vi "ReadSpectrum(SubVI).vi"(8 "Continuous \nStrobe Delay":i32, 11 "Enter the \nInetegration Time":i32) -> (1 "Spectrum Values":dbl[](array[numeric]), 2 "WL Values":dbl[](array[numeric]), 3 "Number of Spectrometers":i32)   [LabVIEW 2022 SP3]
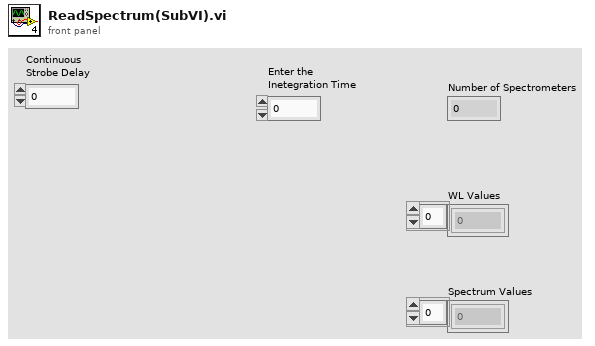
[diagram p1: front panel]
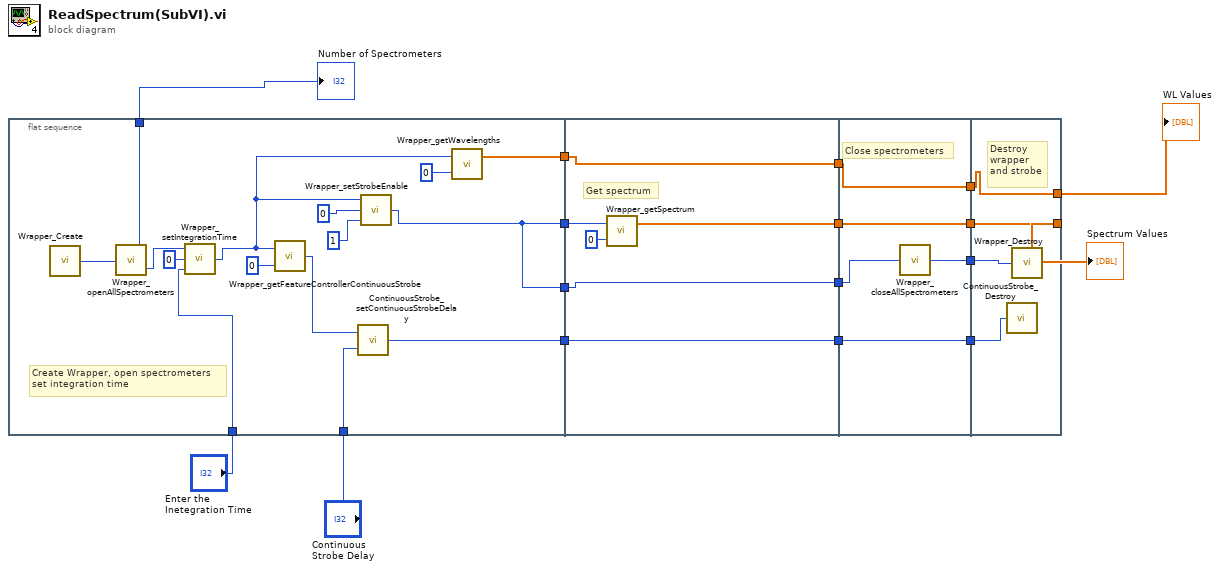
[diagram p0: block diagram]
diagram:
  n1 = flat-sequence {
    tunnel: [w23] -> w17
    tunnel: [w22] -> w16
    tunnel: [w22] -> w15
    tunnel: [w21] -> w14
    tunnel: "Enter the \nInetegration Time" -> [w20]
    tunnel: [w19] -> w5
    tunnel: "Continuous \nStrobe Delay" -> [w18]
    tunnel: [w38] -> w13
    tunnel: w17 -> [w38]
    tunnel: w16 -> [w37]
    tunnel: w15 -> [w35]
    tunnel: [w35] -> w12
    tunnel: w14 -> [w34]
    tunnel: [w34] -> w11
    tunnel: [w33] -> w10
    tunnel: [w43] -> w9
    tunnel: w13 -> [w43]
    tunnel: w12 -> [w42]
    tunnel: [w41] -> w8
    tunnel: [w40] -> w7
    tunnel: w11 -> [w40]
    tunnel: [w39] -> w6
    tunnel: w10 -> [w39]
    tunnel: w9 -> [w47]
    tunnel: w8 -> [w46]
    tunnel: [w45] -> w3
    tunnel: w7 -> [w45]
    tunnel: [w44] -> w2
    tunnel: w6 -> [w44]
    frame #0 {
      # "Create Wrapper, open spectrometers\nset integration time"
      n2 = call "Wrapper_Create.vi"() -> ("Wrapper"=w32:u32)
      n3 = call "Wrapper_openAllSpectrometers.vi"("Wrapper In"=w32) -> ("Number of Spectrometers"=w19:i32, "Wrapper Out"=w26:u32)
      n4 = call "Wrapper_setIntegrationTime.vi"("Integration Time"=w20, "Spectrometer Index"=0 ("Index"), "Wrapper In"=w26) -> ("Wrapper Out"=w24:u32)
      n5 = call "Wrapper_getFeatureControllerContinuousStrobe.vi"("Index"=0, "Wrapper"=w24) -> ("ContinuousStrobe"=w29:u32)
      n6 = call "ContinuousStrobe_setContinuousStrobeDelay.vi"("delay"=w18, "ContinuousStrobe In"=w29) -> ("ContinuousStrobe Out"=w23:u32)
      n7 = call "Wrapper_setStrobeEnable.vi"("On/Off"=1, "Index"=0, "Wrapper In"=w24) -> ("Wrapper Out"=w22:u32)
      n8 = call "Wrapper_getWavelengths.vi"("Index"=0, "Wrapper"=w24) -> ("WL Values"=w21:dbl[])  [unwired: 1 out]
    }
    frame #1 {
      # "Get spectrum"
      n9 = call "Wrapper_getSpectrum.vi"("Index"=0, "Wrapper"=w37) -> ("Spectrum Values"=w33:dbl[])  [unwired: 1 out]
    }
    frame #2 {
      # "Close spectrometers"
      n10 = call "Wrapper_closeAllSpectrometers.vi"("Wrapper In"=w42) -> ("Wrapper Out"=w41:u32)
    }
    frame #3 {
      # "Destroy \nwrapper \nand strobe"
      n11 = call "ContinuousStrobe_Destroy.vi"("ContinuousStrobe"=w47) -> ()
      n12 = call "Wrapper_Destroy.vi"("Wrapper"=w46) -> ()
    }
  }
  "Number of Spectrometers" <- w5
  "Spectrum Values" <- w2
  "WL Values" <- w3
